vi "Get Silent Option.vi"(11 "error in (no error)":errorcluster) -> (4 "Silent Option Enabled?":bool, 15 "error out":errorcluster)   [LabVIEW 2023, in "RFCalAndFixtureCharact.Common.lvlib"]
uses:
  RFCalAndFixtureCharact.Common.lvlib
  Data Cache/Settings Dictionary/Setting Keys.vi
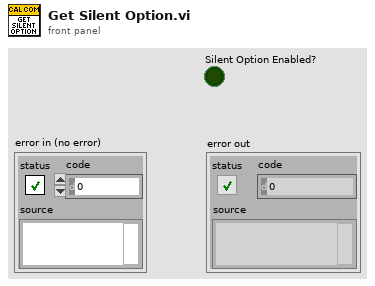
[diagram p1: front panel]
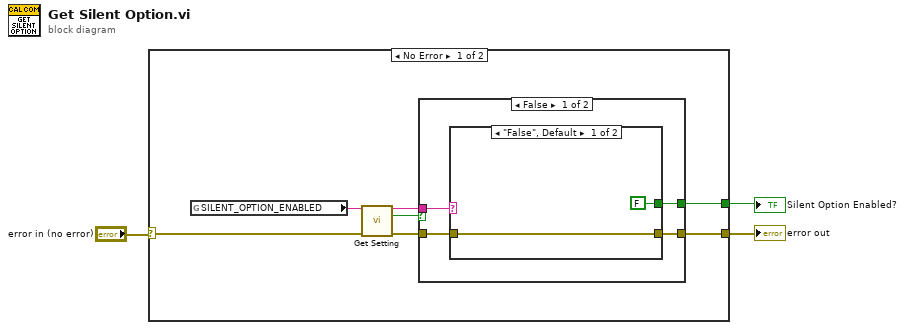
[diagram p0: block diagram]
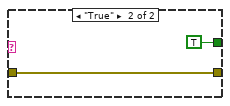
[diagram p2: hidden frame]
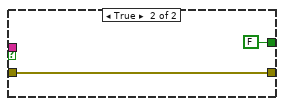
[diagram p3: hidden frame]
diagram:
  n1 = case shown="No Error" "error in (no error)" {
    selector: "error in (no error)" -> [w6 w21]
    tunnel: [w4 w21] -> w2
    tunnel: [w5 _] -> w1
    frame No Error {
      n2 = global read "Setting Keys.vi" "SILENT_OPTION_ENABLED"() -> (w10:string)
      n3 = call "Get Setting.vi"("Setting name"=w10, "error in (no error)"=w6) -> ("Setting value out"=w7:string, "Setting empty or not found?"=w8:bool, "error out"=w9:errorcluster)  [unwired: 11 in]
      n4 = case shown="False" w8 {
        tunnel: [w13 w20] -> w4
        tunnel: w9 -> [w12 w20]
        tunnel: w7 -> [w14 _]
        tunnel: [w11 FALSE] -> w5
        frame False {
          n5 = case shown="\"False\", Default" w14 {
            tunnel: [w16 w18] -> w13
            tunnel: w12 -> [w16 w18]
            tunnel: [FALSE TRUE] -> w11
            frame "False", Default {
            }
            frame "True" {
            }
          }
        }
        frame True {
        }
      }
    }
    frame Error {
    }
  }
  "error out" <- w2
  "Silent Option Enabled?" <- w1
